vi "数据解析.vi"(15 "data in":string) -> (0 "内容说明":string, 1 "内容标识":string, 2 "时标":string, 3 "帧头":string, 5 "帧数":string, 7 "帧号":string, 8 "data out":string, 9 "帧长":string, 10 "CRC":string, 11 "帧内容":string, 13 "结束标志":string)   [LabVIEW 2016, in "数据传输系统-02.lvlib" / "自动更新.lvlib" / "TCP文件传输系统.lvlib" / "TCP发送文件.lvlib"]
panel:
  out "长度 3":i32
  out "长度 2":i32
  out "长度":i32
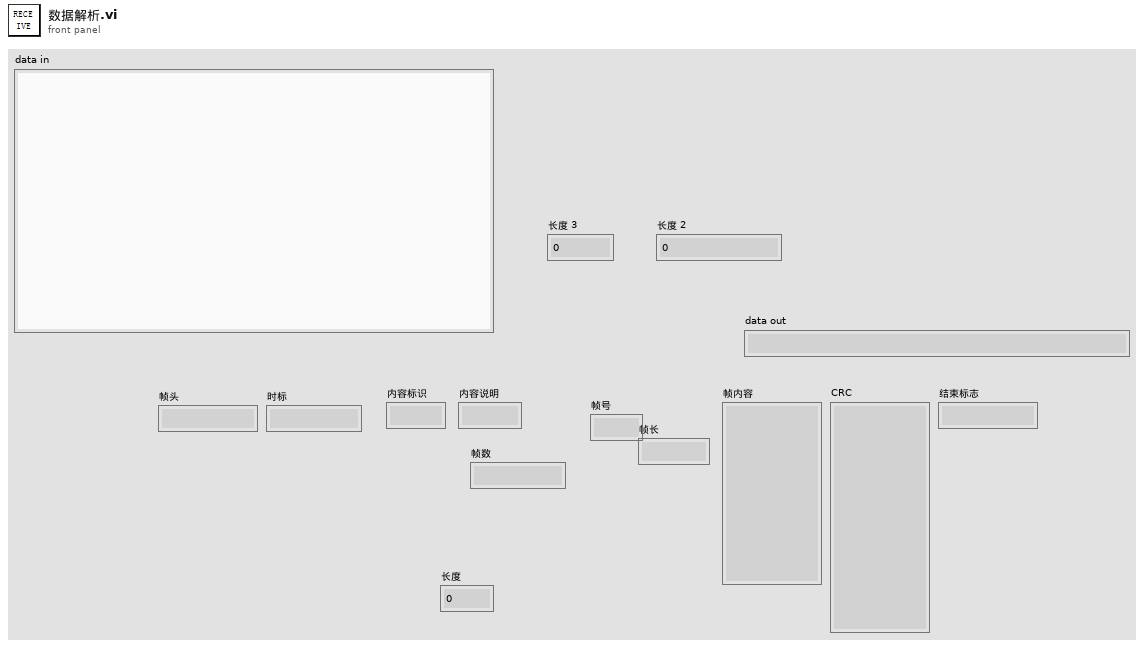
[diagram p1: front panel]
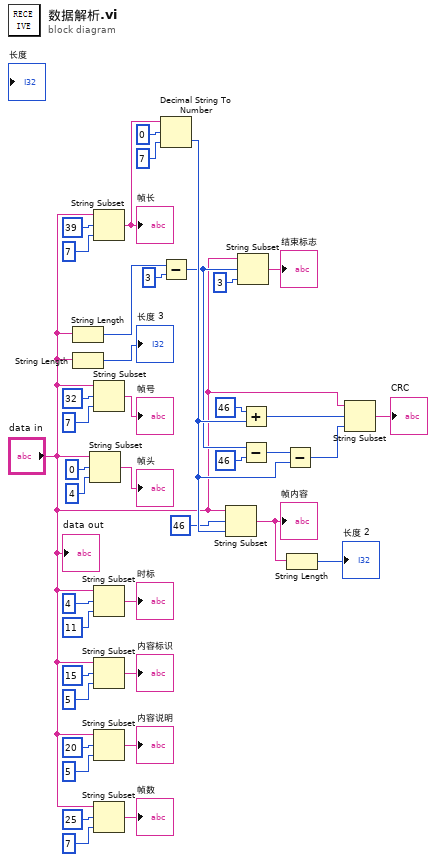
[diagram p0: block diagram]
diagram:
  n1 = String Length(string="data in") -> (length=w38:i32)
  n2 = String Length(string="data in") -> (length=→"长度 3":i32)
  n3 = String Subset(string="data in", offset (0)=0 ("偏移量(0)"), length (rest)=4 ("长度（剩余）")) -> (substring=→"帧头":string)
  n4 = String Subset(string="data in", offset (0)=39 ("偏移量(0)"), length (rest)=7 ("长度（剩余）")) -> (substring=w30:string)
  "帧长" <- w30
  n5 = String Subset(string="data in", offset (0)=32 ("偏移量(0)"), length (rest)=7 ("长度（剩余）")) -> (substring=→"帧号":string)
  n6 = String Subset(string="data in", offset (0)=4 ("偏移量(0)"), length (rest)=11 ("长度（剩余）")) -> (substring=→"时标":string)
  n7 = String Subset(string="data in", offset (0)=15 ("偏移量(0)"), length (rest)=5 ("长度（剩余）")) -> (substring=→"内容标识":string)
  n8 = String Subset(string="data in", offset (0)=20 ("偏移量(0)"), length (rest)=5 ("长度（剩余）")) -> (substring=→"内容说明":string)
  n9 = String Subset(string="data in", offset (0)=25 ("偏移量(0)"), length (rest)=7 ("长度（剩余）")) -> (substring=→"帧数":string)
  n10 = Decimal String To Number(string=w30, offset=0 ("偏移量"), default (0L)=7 ("默认(0 I32)")) -> (number=w36:i32)  [unwired: 1 out]
  n11 = Subtract(x=w38, y=3) -> (x-y=w9:i32)
  n12 = String Subset(string="data in", offset (0)=46 ("偏移量(0)"), length (rest)=w36) -> (substring=w4:string)
  "帧内容" <- w4
  n13 = String Subset(string="data in", offset (0)=w9, length (rest)=3 ("长度（剩余）")) -> (substring=→"结束标志":string)
  n14 = Add(x=46 ("偏移量(0)"), y=w36) -> (x+y=w8:i32)
  n15 = Subtract(x=w9, y=46) -> (x-y=w33:i32)
  n16 = Subtract(x=w33, y=w36) -> (x-y=w7:i32)
  n17 = String Length(string=w4) -> (length=→"长度 2":i32)
  n18 = String Subset(string="data in", offset (0)=w8, length (rest)=w7) -> (substring=→"CRC":string)
  "data out" <- "data in"
